vi "Get Port Number.vi"(8 "error in":errorcluster, 11 "port ref in":T1 format="%.0x") -> (0 "error out":errorcluster, 2 "port number":u16, 3 "port ref out":T1 format="%.0x", 4 "found?":bool)   [LabVIEW 2020, in "ARINC 429 Scripting.lvlib"]
uses:
  ARINC 429 Scripting.lvlib
  <vilib>/NI VeriStand/Custom Device API/Custom Device Item Ref.ctl
  AIM/Constants.vi
  <vilib>/NI VeriStand/Custom Device API/Get Item Property (U16).vi
  <vilib>/NI VeriStand/Custom Device API/Custom Device API.lvlib
  AIM/AIM ARINC 429 Scripting.lvlib
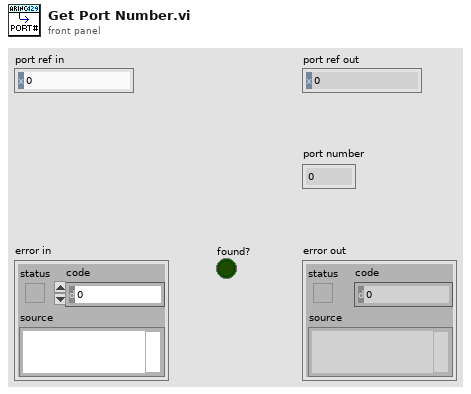
[diagram p1: front panel]
types:
  T1 = typedef "Custom Device API.lvlib/Custom Device Item Ref.ctl" = u64
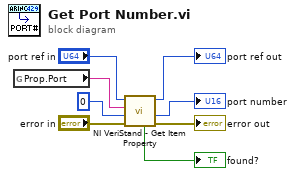
[diagram p0: block diagram]
diagram:
  n1 = global read "Constants.vi" "Prop.Port"() -> (w2:string)
  n2 = call-poly <vilib>:"NI VeriStand - Get Item Property.vi"("error in (no error)"="error in", "Default Value"=u16 0, "Property Name"=w2, "Item Ref in"="port ref in") -> ("error out"=→"error out":errorcluster, "Value"=→"port number":u16, "Item Ref out"=→"port ref out":T1, "Found?"=→"found?":bool)  [unwired: 4 in]
